vi "CleanUp.vi"(8 "error in (no error)":errorcluster, 11 "object in":refnum<class "Wait Monitor.lvclass">) -> (0 "error out":errorcluster, 3 "object out":refnum<class "Wait Monitor.lvclass">)   [LabVIEW 2023, in "HardwareAbstractionLayer_LVOOP.lvlib" / "Wait Monitor.lvclass"]
uses:
  Wait Monitor.lvclass
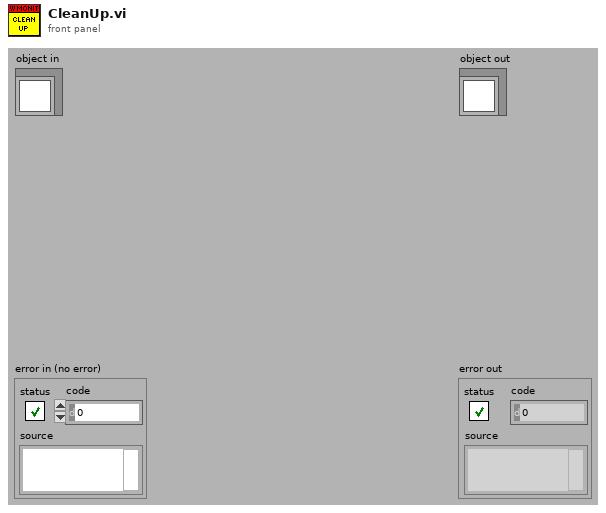
[diagram p1: front panel]
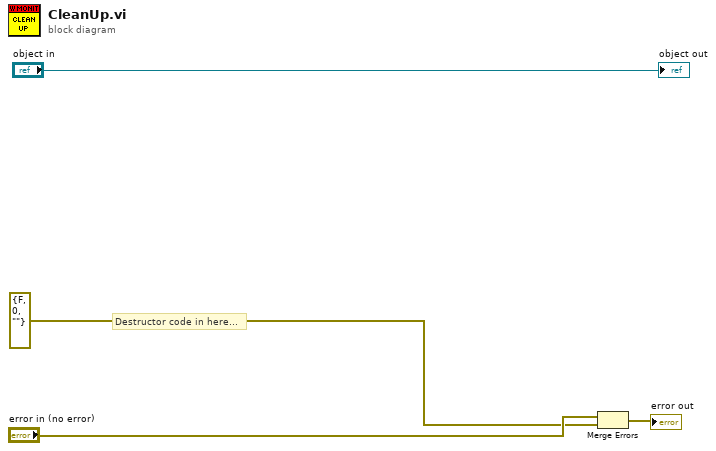
[diagram p0: block diagram]
diagram:
  # "Destructor code in here..."
  n1 = Merge Errors("error in (no error)", errorcluster {"status"=FALSE, "code"=0, "source"=""} ("error in (no error)")) -> (→"error out":errorcluster)
  "object out" <- "object in"
